vi "Demoduler FM_spectre dB.vi"() -> ()   [LabVIEW 2015]
uses:
  <instrlib>/niUSRP/niUSRP Fetch Rx Data (CDB Cluster).vi
  <vilib>/measure/maspectr.llb/FFT Power Spectrum and PSD for 1 Chan.vi
  <vilib>/measure/NI_MAPro.lvlib
  <vilib>/addons/Modulation/niAMT.lvlib
panel:
  out "IQ Plot":waveform(dbl)[](graph)=[{"t0"=timestamp(1136086432.9061224 s since 1904-01-01), "dt"=5e-06, "Y"=array[10000 elements]}, {"t0"=timestamp(1136086432.9061224 s since 1904-01-01), "dt"=5e-06, "Y"=array[10000 elements]}]
  in  "Stop Button":bool
  out "Frequency Plot":cluster{"f0":dbl, "df":dbl, "magnitude":dbl[]}(graph)={"f0"=0.0, "df"=20.0, "magnitude"=array[5000 elements]}
  in  "device names":refnum<k15>="192.168.10.2"
  in  "active antenna":string="RX1"
  in  "number of samples":i64=10000
  out "error out":errorcluster
  out "coerced gain":dbl=10.0 format="%#_6f"
  out "coerced carrier frequency":dbl=95700000.0 format="%#_6p"
  out "coerced IQ rate":dbl=200000.0 format="%#_6p"
  in  "gain":dbl=10.0 format="%#_6f"
  in  "carrier frequency":dbl=95700000.0 format="%#_6p"
  in  "IQ rate":dbl=200000.0 format="%#_6p"
  # "IQ Receiver"
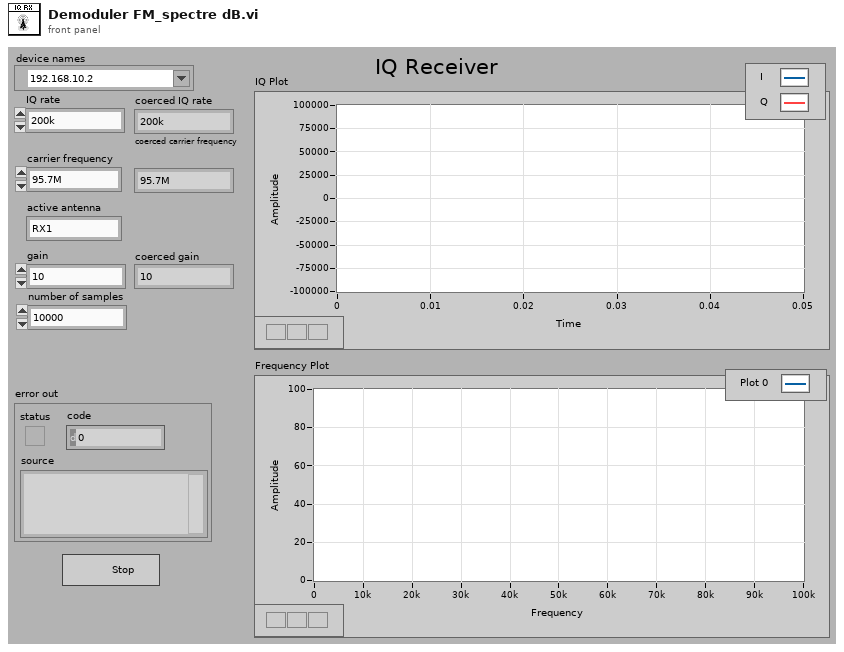
[diagram p1: front panel]
types:
  T1 = typedef "Sound Output Task ID.ctl" = u32
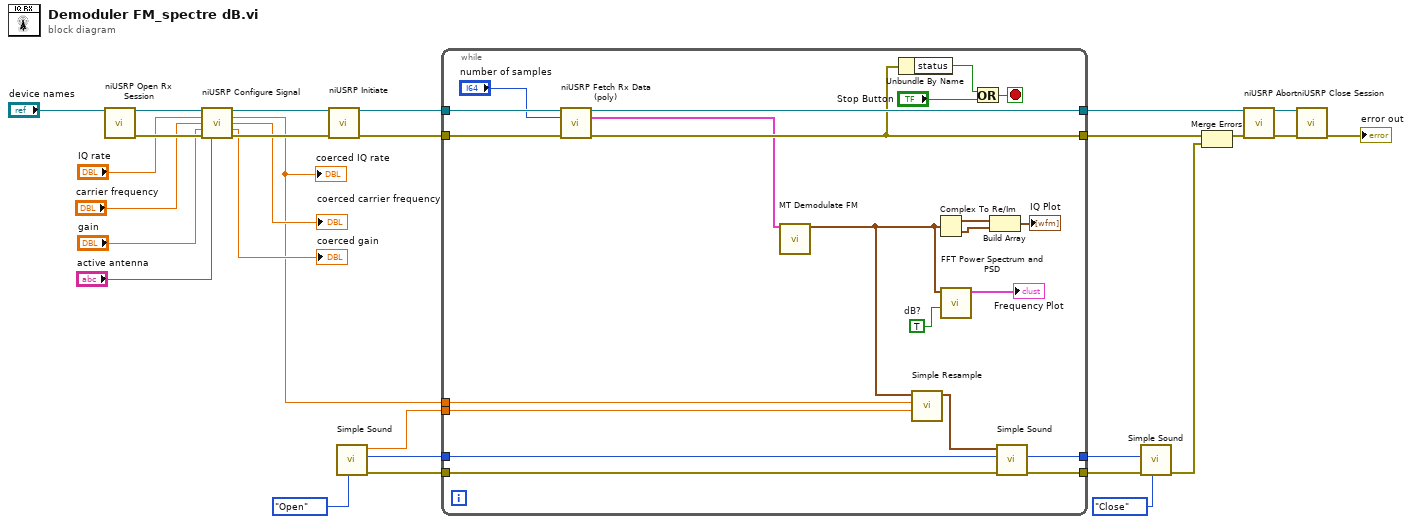
[diagram p0: block diagram]
diagram:
  n1 = call <instrlib>:"niUSRP Open Rx Session.vi"("device names"="device names") -> ("session handle out"=w27:refnum<k15>, "error out"=w26:errorcluster)  [unwired: 13 in]
  n2 = call <instrlib>:"niUSRP Configure Signal.vi"("session handle"=w27, "IQ rate"="IQ rate", "carrier frequency"="carrier frequency", "gain"="gain", "error in (no error)"=w26, "active antenna"="active antenna") -> ("session handle out"=w16:refnum<k15>, "coerced IQ rate"=w5:dbl, "coerced carrier frequency"=→"coerced carrier frequency":dbl, "coerced gain"=→"coerced gain":dbl, "error out"=w18:errorcluster)  [unwired: 5 in]
  "coerced IQ rate" <- w5
  n3 = call <instrlib>:"niUSRP Initiate.vi"("session handle"=w16, "error in (no error)"=w18) -> ("session handle out"=w22:refnum<k15>, "error out"=w21:errorcluster)  [unwired: 12 in]
  n4 = call "Simple Sound.vi"("Action"=enum16{"Open", "Write", "Close"}."Open") -> ("error out"=w3:errorcluster, "task ID out"=w4:T1, "sample rate (S/s)"=w6:dbl)  [unwired: 6 in]
  n5 = while {
    tunnel: w22 -> [w50]
    tunnel: w21 -> [w49]
    tunnel: [w45] -> w12
    tunnel: [w44] -> w10
    tunnel: w6 -> [w40]
    tunnel: w5 -> [w39]
    tunnel: w4 -> [w32]
    tunnel: w3 -> [w31]
    tunnel: [w35] -> w2
    tunnel: [w34] -> w1
    stop <- w43 stop-if-true
    w46 = TRUE  # dB?
    n6 = call-poly <instrlib>:"niUSRP Fetch Rx Data (poly).vi"("session handle"=w50, "number of samples"="number of samples", "error in (no error)"=w49) -> ("session handle out"=w45:refnum<k15>, "data"=w30:cluster{"t0":dbl, "dt":dbl, "Y":cdb[]}, "error out"=w44:errorcluster)  [unwired: 9 in, 1 out]
    n7 = call <vilib>:"MT Demodulate FM.vi"("FM modulated waveform"=w30) -> ("FM demodulated waveform"=w29:waveform(dbl))  [unwired: 12 in, 2 out]
    n8 = Unbundle By Name(w44) -> ("status"=w48:bool)
    n9 = call "Simple Resample.vi"("sample rate (S/s)"=w40, "coerced IQ Rate"=w39, "input waveform"=w29) -> ("output waveform"=w33:waveform(dbl))  [unwired: 8 in]
    n10 = Complex To Re/Im(x + iy=w29) -> (x=w38:waveform(dbl), y=w37:waveform(dbl))
    n11 = call-poly <vilib>:"FFT Power Spectrum and PSD.vi"("dB On (F)"=w46, "time signal"=w29) -> ("Power Spectrum / PSD"=→"Frequency Plot":cluster{"f0":dbl, "df":dbl, "magnitude":dbl[]})  [unwired: 6 in, 3 out]
    n12 = Or(x=w48, y="Stop Button") -> (x .or. y?=w43:bool)
    n13 = Build Array(w38, w37) -> (→"IQ Plot":waveform(dbl)[])
    n14 = call "Simple Sound.vi"("error in"=w31, "task ID"=w32, "data"=w33) -> ("error out"=w35:errorcluster, "task ID out"=w34:T1)  [unwired: 4 in, 1 out]
  }
  n15 = call "Simple Sound.vi"("Action"=enum16{"Open", "Write", "Close"}."Close", "error in"=w2, "task ID"=w1) -> ("error out"=w7:errorcluster)  [unwired: 4 in, 2 out]
  n16 = Merge Errors "Merge Errors"(w10, w7) -> (w9:errorcluster)
  n17 = call <instrlib>:"niUSRP Abort.vi"("session handle"=w12, "error in (no error)"=w9) -> ("session handle out"=w24:refnum<k15>, "error out"=w23:errorcluster)  [unwired: 12 in]
  n18 = call <instrlib>:"niUSRP Close Session.vi"("session handle"=w24, "error in (no error)"=w23) -> ("error out"=→"error out":errorcluster)  [unwired: 13 in]
